vi "Write Control Mode.vi"(8 "error in":errorcluster, 10 "Control Mode":T1 items=["Bus/RS232"=0, "FLOW-BUS slave"=2, "Valve close"=3, "Controller idle"=4, "Setpoint 100%"=7, "Valve fully open"=8, "Calibration mode"=9, "Setpoint 0%"=12, "RS232"=18, "Valve steering"=20, "Valve safe state"=22], 11 "MB_TCP session in":refnum<class "MB_Master_TCP.lvclass">) -> (0 "error out":errorcluster, 3 "MB session out":refnum<class "MB_Master_TCP.lvclass">)   [LabVIEW 2024, in "Bronkhorst Flexi-Flow ModbusTCP API.lvlib"]
uses:
  Bronkhorst Flexi-Flow ModbusTCP API.lvlib
  <vilib>/Plasmionique/MB Master/MB_Master_TCP/MB_Master_TCP.lvclass
  Control Mode--enum.ctl
  PDU Address Char 8-bit Params--ring.ctl
  Write Char Register.vi
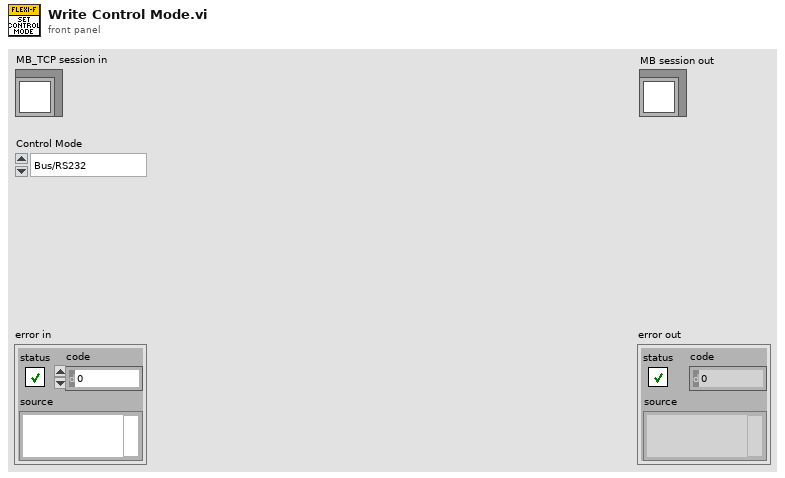
[diagram p1: front panel]
types:
  T1 = typedef "Bronkhorst Flexi-Flow ModbusTCP API.lvlib/Control Mode--enum.ctl" = u16
  T2 = typedef "Bronkhorst Flexi-Flow ModbusTCP API.lvlib/PDU Address Char 8-bit Params--ring.ctl" = u16
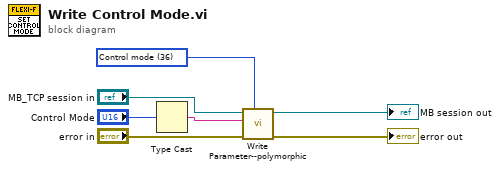
[diagram p0: block diagram]
diagram:
  w3 = T2 36 items=["Wink"=0, "Control mode"=36, "Alarm mode"=3107, "Alarm setpoint"=3109, "Reset alarm enable"=3113, "Counter setpoint mode"=3333, "Reset counter enable"=3337, "Modbus slave address"=4010] ("PDU Address Char 8-bit")
  n1 = Type Cast(x="Control Mode") -> (*(type *) &x=w1:string)  [unwired: 1 in]
  n2 = call-poly "Write Parameter--polymorphic.vi"("PDU Address Char 8-bit"=w3, "error in"="error in", "Unsigned Char"=w1, "MB_TCP session in"="MB_TCP session in") -> ("error out"=→"error out":errorcluster, "MB session out"=→"MB session out":refnum<class "MB_Master_TCP.lvclass">)  [unwired: 6 in]
